vi "Collect_All_Tracks_in_Array-1.vi"(2 "error in":errorcluster, 3 "Tracks(Frames) #2":dbl[][](array[numeric]), 4 "Tracks(Frames) #1":dbl[][](array[numeric])) -> (0 "error out":errorcluster, 1 "[OUT] Collected Tracks":dbl[][](array[numeric]))   [LabVIEW 2013]
doc: "Merges displacement from 2 sources in 1 array"
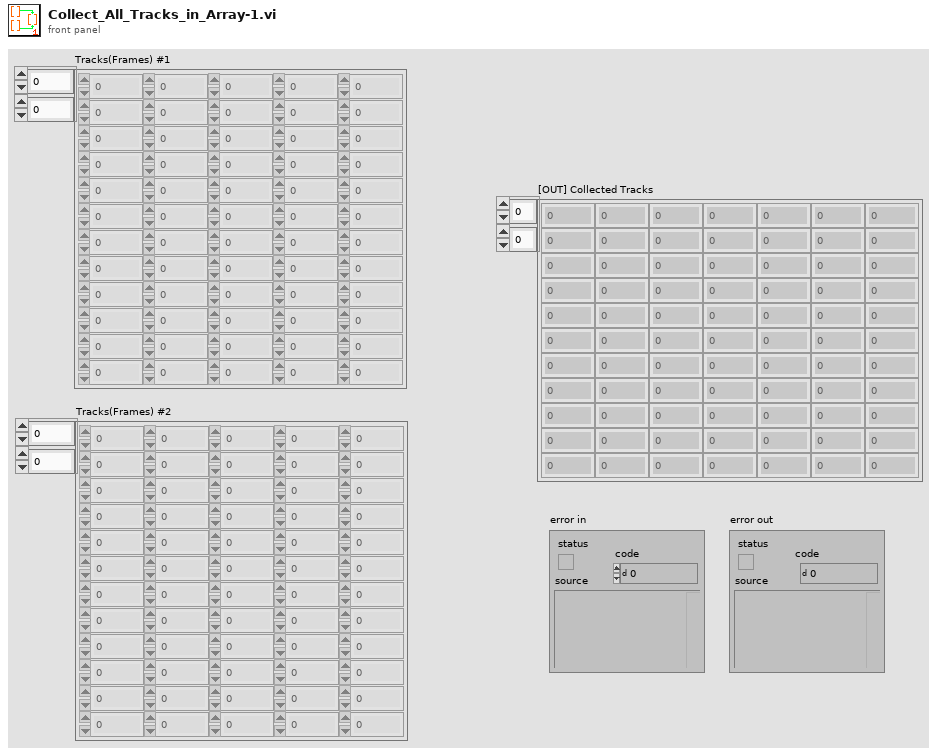
[diagram p1: front panel]
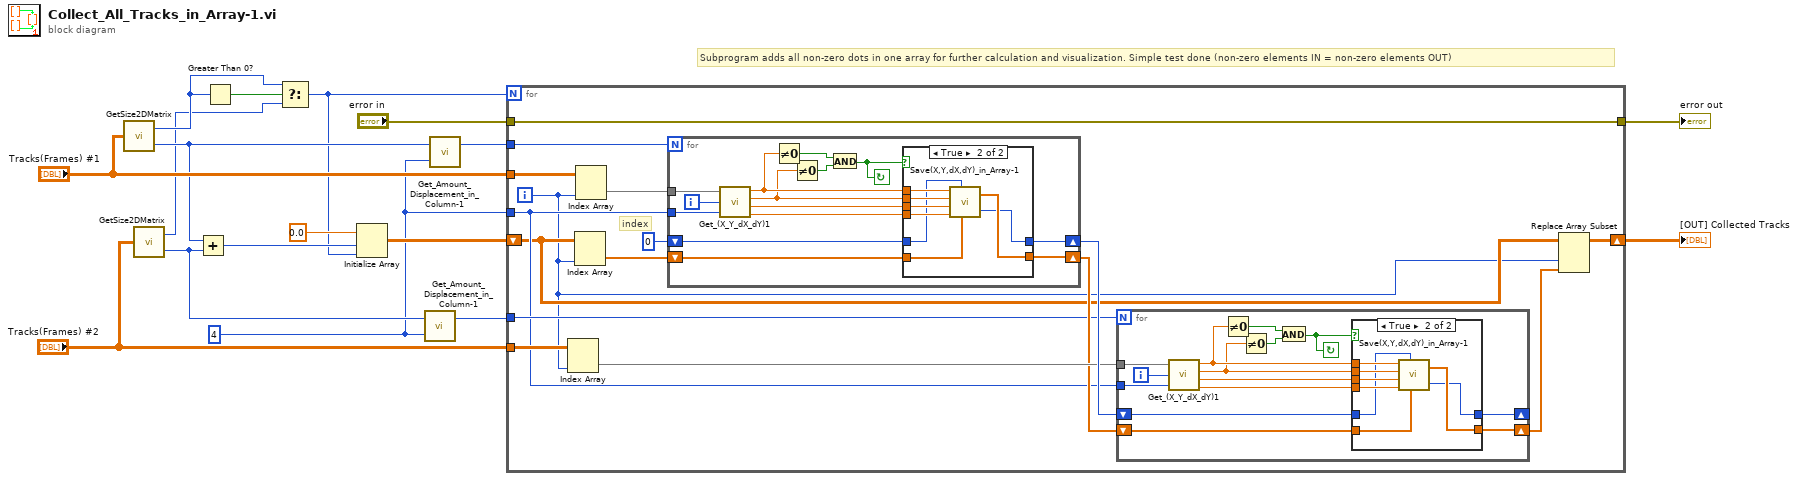
[diagram p0: block diagram]
diagram:
  w8 = 4 ("y")
  # "Subprogram adds all non-zero dots in one array for further calculation and visualization. Simple test done (non-zero elements IN = non-zero elements OUT)"
  n1 = call "GetSize2DMatrix.vi"("Array IN (2D)"="Tracks(Frames) #1") -> ("# Cols"=w5:i32, "# Rows"=w9:i32)
  n2 = call "GetSize2DMatrix.vi"("Array IN (2D)"="Tracks(Frames) #2") -> ("# Cols"=w4:i32, "# Rows"=w11:i32)
  n3 = Add(x=w9, y=w11) -> (x+y=w17:i32)
  n4 = Greater Than 0?(x=w5) -> (x > 0?=w6:bool)
  n5 = Select(t=w5, s=w6, f=w4) -> (s? t:f=w3:i32)
  n6 = Initialize Array(0.0 ("element"), w17, w3) -> (w15:dbl[][])
  n7 = call "Get_Amount_Displacement_in_Column-1.vi"("multiplier"=w8, "# Rows"=w11) -> ("Displ amount"=w10:i32)  [unwired: 1 out]
  n8 = call "Get_Amount_Displacement_in_Column-1.vi"("multiplier"=w8, "# Rows"=w9) -> ("Displ amount"=w7:i32)  [unwired: 1 out]
  n9 = for {
    N: w3 -> [_]
    tunnel: "Tracks(Frames) #1" -> [w33]
    shift-right: [w19] -> w12
    shift-left: w15 -> [w22]
    tunnel: "Tracks(Frames) #2" -> [w29]
    tunnel: w7 -> [w26]
    tunnel: w8 -> [w23]
    tunnel: w10 -> [w24]
    tunnel: "error in" -> [w18]
    tunnel: [w18] -> w1
    i -> [w20]
    # "index"
    n10 = Index Array(array=w29, index (col)=w20) -> (element=w27:dbl[])  [unwired: 1 in]
    n11 = Index Array(array=w22, index (col)=w20) -> (element=w31:dbl[])  [unwired: 1 in]
    n12 = Index Array(array=w33, index (col)=w20) -> (element=w32:dbl[])  [unwired: 1 in]
    n13 = for {
      N: w26 -> [_]
      tunnel: w32 -> [w71]
      tunnel: w23 -> [w69]
      shift-right: [w58] -> w25
      shift-left: w31 -> [w60]
      shift-right: [w59] -> w28
      shift-left: 0 -> [w61]
      i -> [w70]
      stop <- w66 continue-if-true
      n14 = call "Get_(X_Y_dX_dY)1.vi"("(X,Y,dX,dY)"=w71, "index"=w70, "multiplier"=w69) -> ("X"=w65:dbl, "Y"=w64:dbl, "dX"=w63:dbl, "dY"=w62:dbl)
      n15 = Not Equal To 0?(x=w65) -> (x != 0?=w68:bool)
      n16 = Not Equal To 0?(x=w64) -> (x != 0?=w67:bool)
      n17 = And(x=w68, y=w67) -> (x .and. y?=w66:bool)
      n18 = case shown="True" w66 {
        tunnel: w65 -> [_ w81]
        tunnel: w64 -> [_ w80]
        tunnel: w63 -> [_ w79]
        tunnel: w62 -> [_ w78]
        tunnel: w61 -> [w72 w77]
        tunnel: w60 -> [w73 w76]
        tunnel: [w73 w75] -> w58
        tunnel: [w72 w74] -> w59
        frame False {
        }
        frame True {
          n19 = call "Save(X,Y,dX,dY)_in_Array-1.vi"("Array for Replacement IN"=w76, "Starting Position"=w77, "dY"=w78, "dX"=w79, "Y"=w80, "X"=w81) -> ("Finish Position"=w74:i32, "Array for Replacement OUT"=w75:dbl[])
        }
      }
    }
    n20 = for {
      N: w24 -> [_]
      tunnel: w27 -> [w47]
      tunnel: w23 -> [w45]
      shift-right: [w34] -> w21
      shift-left: w25 -> [w36]
      shift-right: [w35] -> _
      shift-left: w28 -> [w37]
      i -> [w46]
      stop <- w42 continue-if-true
      n21 = call "Get_(X_Y_dX_dY)1.vi"("(X,Y,dX,dY)"=w47, "index"=w46, "multiplier"=w45) -> ("X"=w41:dbl, "Y"=w40:dbl, "dX"=w39:dbl, "dY"=w38:dbl)
      n22 = Not Equal To 0?(x=w41) -> (x != 0?=w44:bool)
      n23 = Not Equal To 0?(x=w40) -> (x != 0?=w43:bool)
      n24 = And(x=w44, y=w43) -> (x .and. y?=w42:bool)
      n25 = case shown="True" w42 {
        tunnel: w41 -> [_ w57]
        tunnel: w40 -> [_ w56]
        tunnel: w39 -> [_ w55]
        tunnel: w38 -> [_ w54]
        tunnel: w37 -> [w48 w53]
        tunnel: w36 -> [w49 w52]
        tunnel: [w49 w51] -> w34
        tunnel: [w48 w50] -> w35
        frame False {
        }
        frame True {
          n26 = call "Save(X,Y,dX,dY)_in_Array-1.vi"("Array for Replacement IN"=w52, "Starting Position"=w53, "dY"=w54, "dX"=w55, "Y"=w56, "X"=w57) -> ("Finish Position"=w50:i32, "Array for Replacement OUT"=w51:dbl[])
        }
      }
    }
    n27 = Replace Array Subset(array=w22, new element=w21, index (col)=w20) -> (w19:dbl[][])  [unwired: 1 in]
  }
  "[OUT] Collected Tracks" <- w12
  "error out" <- w1
